vi "Focus.vi"(8 "error in (no error)":errorcluster, 11 "LightField Automation in":refnum<class "LightField Automation.lvclass">) -> (0 "error out":errorcluster, 3 "LightField Automation out":refnum<class "LightField Automation.lvclass">)   [LabVIEW 2015]
uses:
  LightField Automation.lvclass
  C:/Program Files/Princeton Instruments/LightField/AddInViews/PrincetonInstruments.LightFieldViewV3.dll
  Program Files/Princeton Instruments/LightField/AddInViews/PrincetonInstruments.LightFieldViewV3.dll
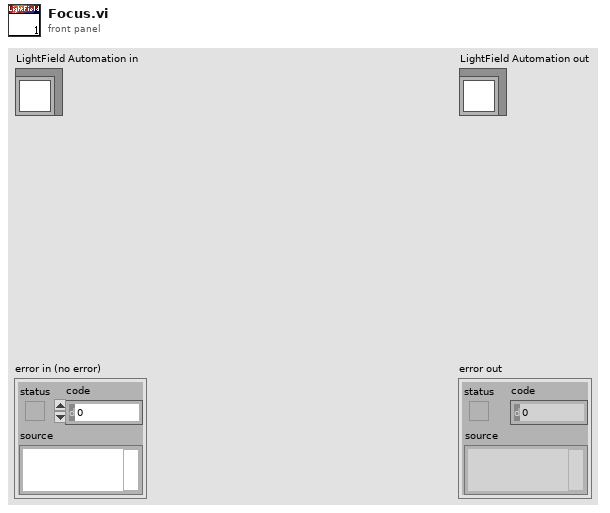
[diagram p1: front panel]
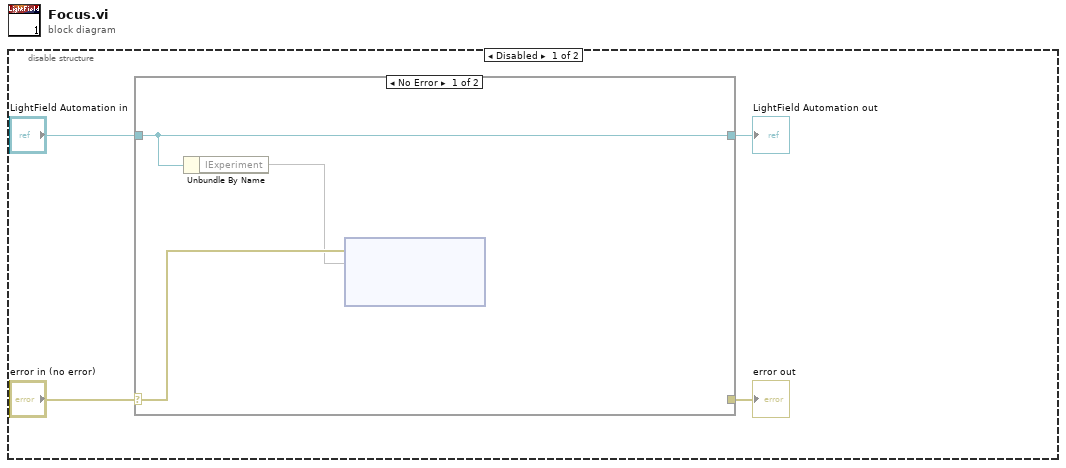
[diagram p0: block diagram]
diagram:
  n1 = disable-structure shown="Disabled" {
    frame Disabled {
      n2 = case shown="No Error" "error in (no error)" {
        selector: "error in (no error)" -> [w6 w9]
        tunnel: [_ w9] -> w3
        tunnel: [w7 w8] -> w1
        tunnel: "LightField Automation in" -> [w7 w8]
        frame No Error {
          n3 = Unbundle By Name(w7) -> ("IExperiment"=w5)
          n4 = node(w6, w5) -> ()  [unwired: 3 in, 2 out]
        }
        frame Error {
        }
      }
      "error out" <- w3
      "LightField Automation out" <- w1
    }
    frame Enabled {
    }
  }
